vi "Init.vi"(7 "Sender":refnum<class "Sender.lvclass">, 10 "Pump State":bool) -> (3 "Update Pump State Msg out":refnum<class "Update Pump State Msg.lvclass">)   [LabVIEW 2025, in "Update Pump State Msg.lvlib" / "Update Pump State Msg.lvclass"]
uses:
  Update Pump State Msg.lvclass
  <vilib>/Nathan Davis/jettl/jettl/jettl/Sender/Sender/Sender.lvclass
  Update Pump State Msg.lvclass/Update Pump State Msg.ctl
panel:
  # "This front panel should not be manipulated."
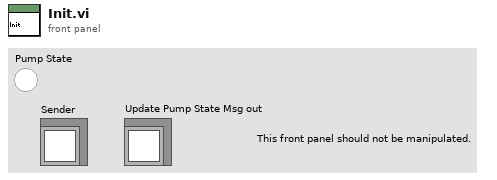
[diagram p1: front panel]
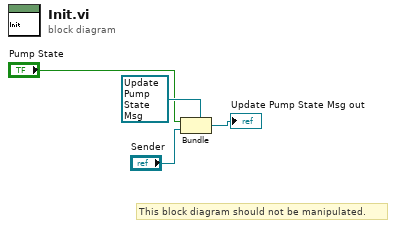
[diagram p0: block diagram]
diagram:
  # "This block diagram should not be manipulated."
  n1 = Bundle "Bundle"(cluster=refnum<class "Update Pump State Msg.lvclass"> refnum ("TEMPLATE Msg Strategy out"), "Pump State", "Sender") -> (→"Update Pump State Msg out":refnum<class "Update Pump State Msg.lvclass">)
